vi "Get Number New Images.vi"(8 "error in (no error)":errorcluster, 11 "CCDCamera in":refnum<class "CCDCamera.lvclass">) -> (0 "error out":errorcluster, 2 "New Images ?":bool, 3 "CCDCamera out":refnum<class "CCDCamera.lvclass">)   [LabVIEW 2018, in "CCDCamera.lvclass"]
uses:
  CCDCamera.lvclass
  CCDCamera.lvclass/CCDCamera.ctl
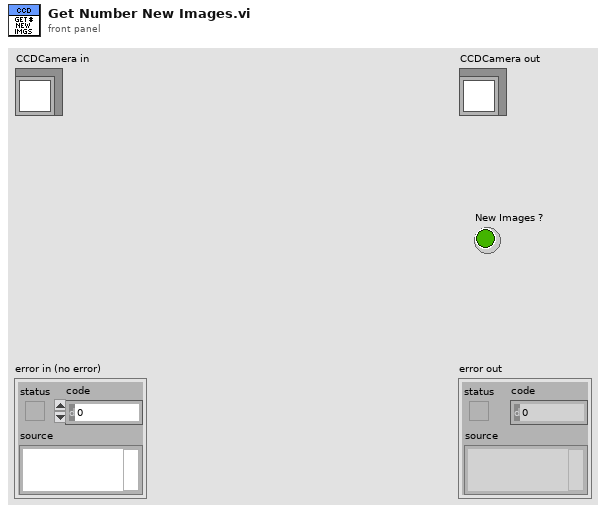
[diagram p1: front panel]
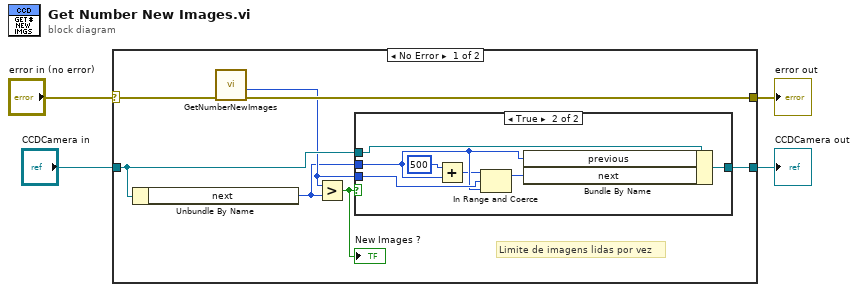
[diagram p0: block diagram]
diagram:
  n1 = case shown="No Error" "error in (no error)" {
    selector: "error in (no error)" -> [w10 w21]
    tunnel: [w11 w21] -> w3
    tunnel: [w9 w20] -> w1
    tunnel: "CCDCamera in" -> [w8 w20]
    frame No Error {
      # "Limite de imagens lidas por vez"
      n2 = Unbundle By Name(w8) -> ("next"=w5:u16)
      n3 = call <userlib>:"GetNumberNewImages.vi"("error in (no error)"=w10) -> ("error out"=w11:errorcluster, "last"=w7:i32)  [unwired: 3 in, 2 out]
      n4 = Greater?(x=w7, y=w5) -> (0:w6:bool)
      "New Images ?" <- w6
      n5 = case shown="True" w6 {
        tunnel: [w12 w19] -> w9
        tunnel: w8 -> [w12 w18]
        tunnel: w7 -> [_ w17]
        tunnel: w5 -> [_ w16]
        frame False {
        }
        frame True {
          n6 = Add(x=u16 500, y=w16) -> (x+y=w15:u16)
          n7 = In Range and Coerce(upper limit=w15, x=w17, lower limit=w16) -> (coerced(x)=w14:i32)  [unwired: 1 out]
          n8 = Bundle By Name(cluster=w18, "previous"=w16, "next"=w14) -> (w19:refnum<class "CCDCamera.lvclass">)
        }
      }
    }
    frame Error {
    }
  }
  "error out" <- w3
  "CCDCamera out" <- w1
